vi "Engine-Delete-Window.vi"(8 "error in (no error)":errorcluster, 11 "Window in":refnum<class "Window.lvclass">) -> (0 "error out":errorcluster)   [LabVIEW 2020, in "GLF.lvlib" / "Window.lvclass"]
uses:
  Window.lvclass
  Window.lvclass/Window.ctl
  IAmGLF/IAmGLF.lvclass
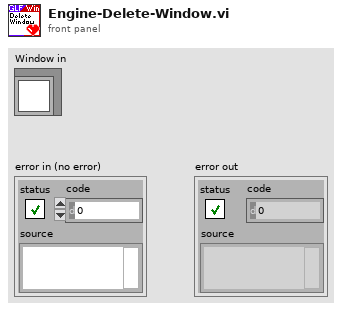
[diagram p1: front panel]
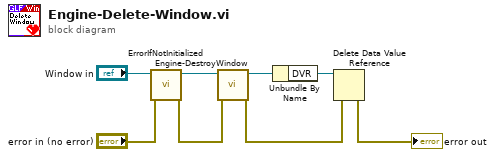
[diagram p0: block diagram]
diagram:
  n1 = call "ErrorIfNotInitialized.vi"("error in (no error)"="error in (no error)", "IAmGLF in"="Window in") -> ("error out"=w7:errorcluster, "IAmGLF out"=w8:refnum<class "Window.lvclass">)  [unwired: 8 in]
  n2 = call "Engine-DestroyWindow.vi"("error in (no error)"=w7, "Window in"=w8) -> ("error out"=w1:errorcluster, "Window out"=w2:refnum<class "Window.lvclass">)  [unwired: 8 in]
  n3 = Unbundle By Name(w2) -> ("DVR"=w3:refnum<data-value>)
  n4 = Delete Data Value Reference(data value reference=w3, error in=w1) -> (error out=→"error out":errorcluster)  [unwired: 1 out]
